vi "Test Get ATM Message when Withdraw Failed.vi"(8 "error in (no error)":errorcluster, 11 "Test Case In":refnum<class "Controller Test.lvclass">) -> (0 "error out":errorcluster, 3 "Test Case Out":refnum<class "Controller Test.lvclass">)   [LabVIEW 2020, in "Controller Test.lvclass"]
uses:
  Controller Test/Controller Test.lvclass
  Controller Test/Controller Test.lvclass/Controller Test.ctl
  01074fa8-ee8a-411d-bc8b-fc92c4f90959.vi
  ATM Controller/ATM Controller.lvclass
  Account Database/Account Data.ctl
  Account Database/Account Database.lvclass
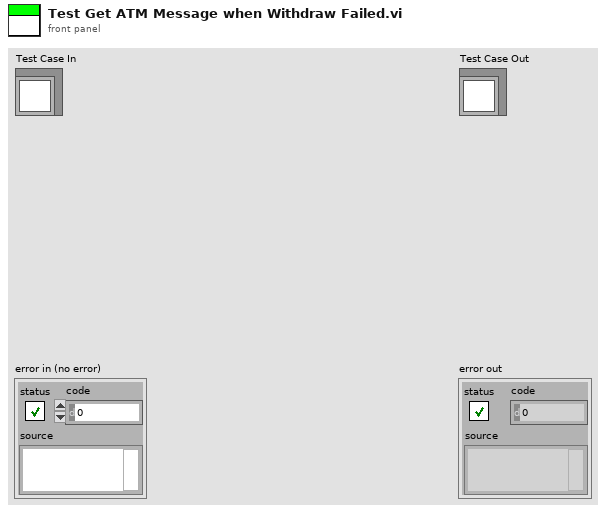
[diagram p1: front panel]
types:
  T1 = typedef "Account Database.lvclass/Account Data.ctl" = cluster{"Account Number":string, "First Name":string, "Last Name":string, "Account Balance":string}
  T2 = typedef "ATM Controller.lvclass/State.ctl" = enum16{"Start", "Card Inserted", "Verification Failed", "Verification Succeeded", "Depositing", "Depositing Completed", "Withdrawing", "Withdraw Completed", "Withdraw Failed", "Terminate"}
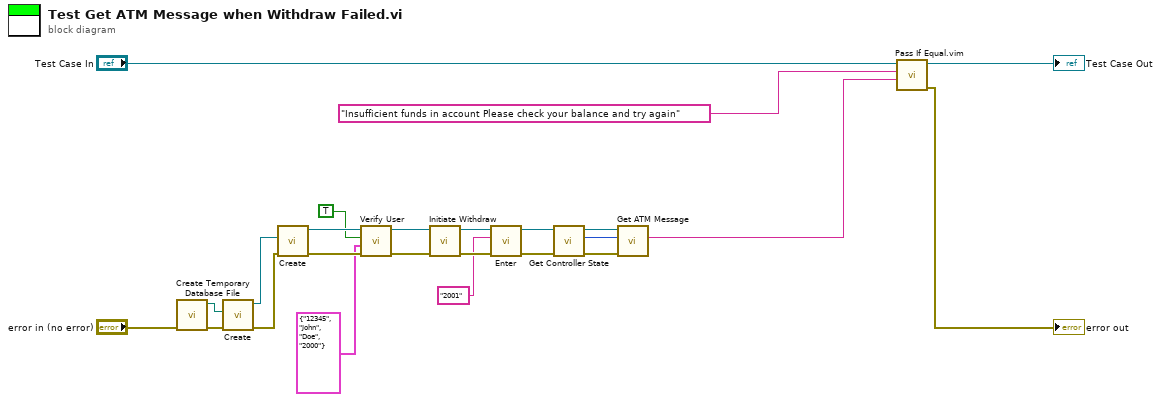
[diagram p0: block diagram]
diagram:
  n1 = call "Create Temporary Database File.vi"("error in (no error)"="error in (no error)") -> ("error out"=w4:errorcluster, "path"=w2:path)  [unwired: 9 in]
  n2 = call "Create.vi"("error in (no error)"=w4, "Data File"=w2) -> ("error out"=w3:errorcluster, "Account Database out"=w1:refnum<class "Account Database.lvclass">)  [unwired: 8 in]
  n3 = call "Create.vi"("error in (no error)"=w3, "Account Database"=w1) -> ("error out"=w20:errorcluster, "ATM Controller out"=w16:refnum<class "ATM Controller.lvclass">)  [unwired: 8 in]
  n4 = call "Verify User.vi"("error in (no error)"=w20, "Account Data"=T1 {"Account Number"="12345", "First Name"="John", "Last Name"="Doe", "Account Balance"="2000"}, "Verified?"=TRUE, "ATM Controller in"=w16) -> ("error out"=w17:errorcluster, "ATM Controller out"=w12:refnum<class "ATM Controller.lvclass">)  [unwired: 6 in]
  n5 = call "Initiate Withdraw.vi"("error in (no error)"=w17, "ATM Controller in"=w12) -> ("error out"=w13:errorcluster, "ATM Controller out"=w10:refnum<class "ATM Controller.lvclass">)  [unwired: 8 in]
  n6 = call "Enter.vi"("error in (no error)"=w13, "User Input"="2001", "ATM Controller in"=w10) -> ("error out"=w11:errorcluster, "ATM Controller out"=w8:refnum<class "ATM Controller.lvclass">)  [unwired: 7 in]
  n7 = call "Get Controller State.vi"("error in (no error)"=w11, "ATM Controller in"=w8) -> ("error out"=w9:errorcluster, "ATM State"=w6:T2, "ATM Controller out"=w7:refnum<class "ATM Controller.lvclass">)  [unwired: 7 in]
  n8 = call "Get ATM Message.vi"("error in (no error)"=w9, "ATM State"=w6, "ATM Controller In"=w7) -> ("Message"=w19:string)  [unwired: 6 in, 2 out]
  n9 = call "Pass If Equal.vim"("Actual"=w19, "Expected"="Insufficient funds in account Please check your balance and try again" ("Message"), "LUnit Test Case In"="Test Case In") -> ("error out"=→"error out":errorcluster, "LUnit Test Case Out"=→"Test Case Out":refnum<class "Controller Test.lvclass">)  [unwired: 7 in]
